vi "[RT] Cont Acq wPause.vi"() -> ()   [LabVIEW 2015]
doc: "If a finite acquisition is too large for the amount of memory available on the host controller, then perform a continuous acquisition for a finite period of time. When you call rwfm_Stop.vi, the FPGA stops the acquisition and immediately rearms itself waiting for rwfm_Start.vi to be called. The stop VI also flushes the host application's data buffer so subsequent acquisitions do not return old data."
uses:
  <vilib>/NI/cRIO Wfm/ChannelConfig.ctl
  <vilib>/FPGAPlugInAG/sbRIO-9607/niLvFpga_Open_sbRIO-9607.vi
  <vilib>/rvi/interface/common/dynamic/niFpgaDynamicAddResources.vi
  <vilib>/FPGAPlugInAG/Dynamic/niLvFpga_Reset_Dynamic.vi
  <vilib>/FPGAPlugInAG/Dynamic/niLvFpga_Run_Dynamic.vi
  <vilib>/FPGAPlugInAG/Dynamic/niLvFpga_Close_Dynamic.vi
  <vilib>/rvi/interface/nirviOpenFPGA/nirviOpenFPGA.xnode
  FPGA Bitfiles/WaveformLibraryI_FPGATarget2_[FPGA]SARAcqMain_U+qOsuK4w1s.lvbitx
  FPGA/[FPGA] SAR Acq Main.vi
  <vilib>/rvi/interface/nirviMethod/nirviMethod.xnode
  <vilib>/rvi/interface/nirviCloseFPGA/nirviCloseFPGA.xnode
  IFw_Addon/RT/WaveformTask.lvclass
  <vilib>/NI/cRIO Wfm/cRIO Wfm.lvlib
panel:
  in  "Sample Rate":u32=51200
  in  "Channel Info":T1=[{"Channel Name"="Mod1/ai0", "Sensitivity mV_EU"=1000.0, "EU"="V", "dB Ref EU"=1.0}, {"Channel Name"="Mod1/ai1", "Sensitivity mV_EU"=1000.0, "EU"="V", "dB Ref EU"=1.0}, {"Channel Name"="Mod1/ai2", "Sensitivity mV_EU"=1000.0, "EU"="V", "dB Ref EU"=1.0}] caption="Channel Name      Scale [mV/EU]        EU           dB Ref [EU]" {"dB Ref EU" format="%#.2p"; "Sensitivity mV_EU" format="%.2f"}
  in  "Samps per Chan":i32=25600 caption="Samples per Channel"
  out "RT Buffer Backlog [%]":dbl format="%#.2g"
  in  "Pause":bool
  out "Waveform Graph":sgl[][](graph)
  in  "stop":bool
  # "Sampling Info"
  # "Channel Info"
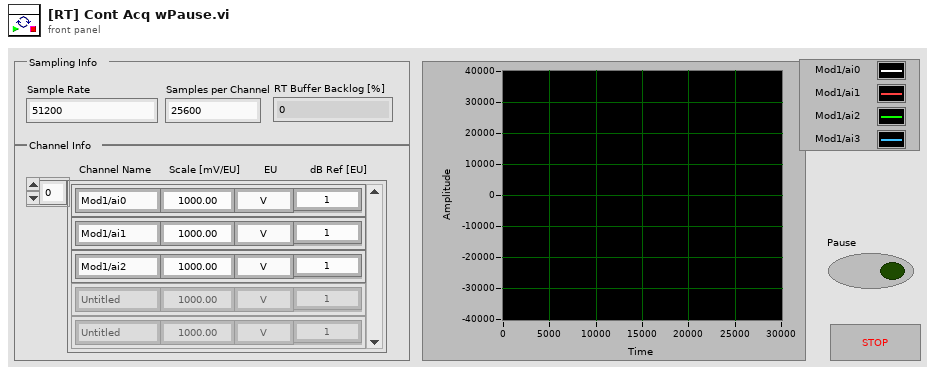
[diagram p1: front panel]
types:
  T1 = typedef "cRIO Wfm.lvlib/ChannelConfig.ctl" = cluster{"Channel Name":string, "Sensitivity mV_EU":dbl, "EU":string, "dB Ref EU":dbl}[]
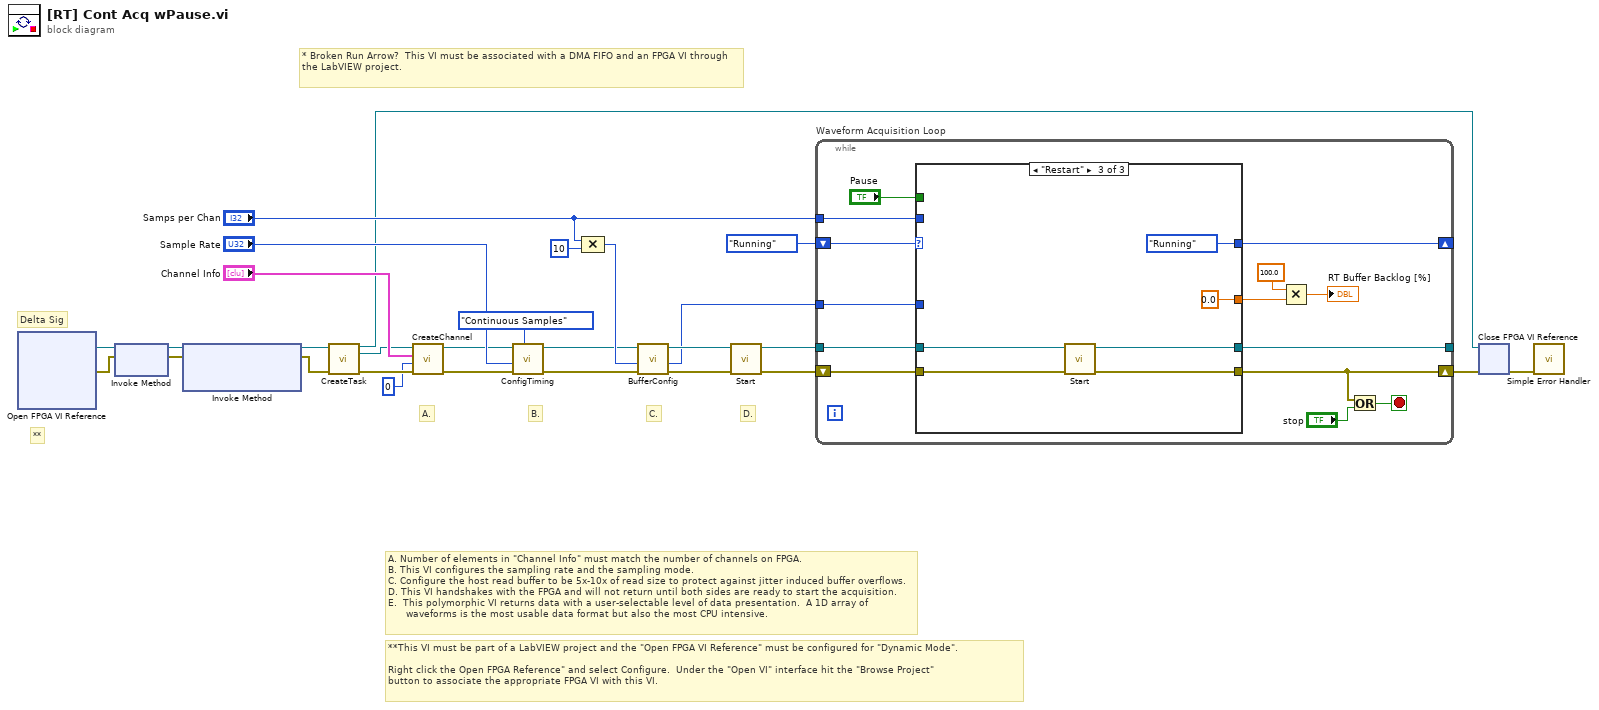
[diagram p0: block diagram]
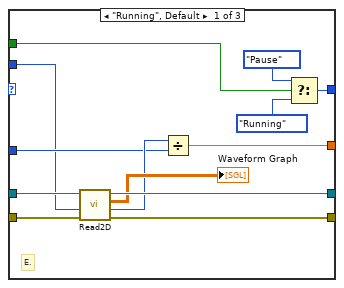
[diagram p2: hidden frame]
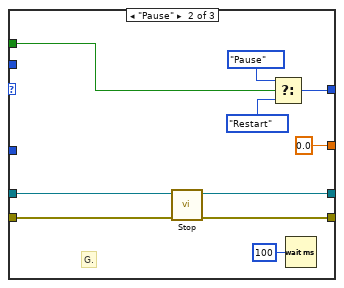
[diagram p3: hidden frame]
diagram:
  # "Delta Sig"
  # "**This VI must be part of a LabVIEW project and the \"Open FPGA VI Reference\" must be configured for \"Dynamic Mode\".\n\nRight click the Open FPGA Reference\" and select Configure.  Under the \"Open VI\" interface hit the \"Browse Project\" \nbutton to associate the appropriate FPGA VI with this VI."
  # "* Broken Run Arrow?  This VI must be associated with a DMA FIFO and an FPGA VI through the LabVIEW project."
  # "**"
  # "D."
  # "C."
  # "B."
  # "A."
  # "A. Number of elements in \"Channel Info\" must match the number of channels on FPGA.\nB. This VI configures the sampling rate and the sampling mode.\nC. Configure the host read buffer to be 5x-10x of read size to protect against jitter induced buffer overflows.\nD. This VI handshakes with the FPGA and will not return until both sides are ready to start the acquisition.\nE.  This polymorphic VI returns data with a user-selectable level of data presentation.  A 1D array of     \n      waveforms is the most usable data format but also the most CPU intensive."
  n1 = xnode "Open FPGA VI Reference"() -> ("FPGA VI Reference Out"=w4:refnum<k20>, "error out"=w3:errorcluster)  [unwired: 2 in]
  n2 = xnode "Invoke Method"("FPGA VI Reference In"=w4, "error in"=w3) -> ("FPGA VI Reference Out"=w6:refnum<k20>, "error out"=w5:errorcluster)
  n3 = xnode "Invoke Method"("FPGA VI Reference In"=w6, "error in"=w5) -> ("FPGA VI Reference Out"=w2:refnum<k20>, "error out"=w1:errorcluster)  [unwired: 1 in]
  n4 = call "CreateTask.vi"("FPGA Ref in"=w2, "error in"=w1) -> ("FPGA Ref out"=w7:refnum<k20>, "Task out"=w15:refnum<class "WaveformTask.lvclass">, "error out"=w16:errorcluster)  [unwired: 11 in]
  n5 = call "CreateChannel.vi"("error in"=w16, "instance"=u8 0, "Channel Info"="Channel Info", "task in"=w15) -> ("error out"=w12:errorcluster, "Task out"=w10:refnum<class "WaveformTask.lvclass">)  [unwired: 6 in]
  n6 = call "ConfigTiming.vi"("Sample Mode"=enum16{"Finite Samples", "Continuous Samples"}."Continuous Samples", "error in (no error)"=w12, "Sample Rate"="Sample Rate", "Task in"=w10) -> ("error out"=w13:errorcluster, "Task out"=w8:refnum<class "WaveformTask.lvclass">)  [unwired: 5 in, 1 out]
  n7 = Compound Arithmetic op=MULTIPLY("Samps per Chan", 10 ("value")) -> (w20:i32)
  n8 = call "BufferConfig.vi"("error in (no error)"=w13, "Buffer Size [Samps per Chan]"=w20, "WaveformTask in"=w8) -> ("error out"=w22:errorcluster, "Buffer Size [Total Samples]"=w19:u32, "WaveformTask out"=w23:refnum<class "WaveformTask.lvclass">)  [unwired: 6 in]
  n9 = call "Start.vi"("error in (no error)"=w22, "WaveformTask in"=w23) -> ("error out"=w27:errorcluster, "WaveformTask out"=w28:refnum<class "WaveformTask.lvclass">)  [unwired: 8 in]
  n10 = while "Waveform Acquisition Loop" {
    tunnel: w28 -> [w41]
    tunnel: [w38] -> _
    shift-right: [w36] -> _
    shift-left: enum16{"Running", "Pause", "Restart"}."Running" ("ReadCmnd") -> [w37]
    tunnel: w19 -> [w34]
    tunnel: "Samps per Chan" -> [w30]
    shift-right: [w29] -> w26
    shift-left: w27 -> [w39]
    stop <- w40 stop-if-true
    n11 = case shown="\"Restart\"" w37 {
      tunnel: w41 -> [w55 w61 w71]
      tunnel: w39 -> [w54 w60 w70]
      tunnel: [w53 w59 w69] -> w38
      tunnel: [w52 w58 w68] -> w29
      tunnel: [w51 w63 enum16{"Running", "Pause", "Restart"}."Running" ("ReadCmnd")] -> w36
      tunnel: "Pause" -> [w48 w62 _]
      tunnel: w34 -> [w45 _ _]
      tunnel: [w44 0.0 0.0] -> w31
      tunnel: w30 -> [w43 _ _]
      frame "Running", Default {
        # "E."
        n12 = call "Read2D.vi"("error in"=w54, "Timeout (s)"=w43, "Task in"=w55) -> ("error out"=w52:errorcluster, "Samples Remaining"=w46:u32, "Data"=→"Waveform Graph":sgl[][], "Task out"=w53:refnum<class "WaveformTask.lvclass">)  [unwired: 5 in]
        n13 = Divide(x=w46, y=w45) -> (x/y=w44:dbl)
        n14 = Select(t=enum16{"Running", "Pause", "Restart"}."Pause" ("ReadCmnd"), s=w48, f=enum16{"Running", "Pause", "Restart"}."Running" ("ReadCmnd")) -> (s? t:f=w51:enum16{"Running", "Pause", "Restart"})
      }
      frame "Pause" {
        # "G."
        n15 = call "Stop.vi"("error in"=w60, "WaveformTask in"=w61) -> ("error out"=w58:errorcluster, "Task out"=w59:refnum<class "WaveformTask.lvclass">)  [unwired: 8 in]
        n16 = Select(t=enum16{"Running", "Pause", "Restart"}."Pause" ("ReadCmnd"), s=w62, f=enum16{"Running", "Pause", "Restart"}."Restart" ("ReadCmnd")) -> (s? t:f=w63:enum16{"Running", "Pause", "Restart"})
        n17 = Wait (ms)(milliseconds to wait=u32 100) -> ()  [unwired: 1 out]
      }
      frame "Restart" {
        n18 = call "Start.vi"("error in (no error)"=w70, "WaveformTask in"=w71) -> ("error out"=w68:errorcluster, "WaveformTask out"=w69:refnum<class "WaveformTask.lvclass">)  [unwired: 8 in]
      }
    }
    n19 = Multiply(x=100.0, y=w31) -> (x*y=→"RT Buffer Backlog [%]":dbl)
    n20 = Or(x=w29, y="stop") -> (x .or. y?=w40:bool)
  }
  n21 = xnode "Close FPGA VI Reference"("FPGA VI Reference In"=w7, "error in"=w26) -> ("error out"=w24:errorcluster)
  n22 = call <vilib>:"Simple Error Handler.vi"("error in (no error)"=w24) -> ()  [unwired: 1 in, 8 out]
